vi "beginning_sound.vi"() -> ()   [LabVIEW 2019]
uses:
  <vilib>/sound2/lvsound2.llb/Sound Data Format.ctl
  <vilib>/sound2/lvsound2.llb/Sampling Mode.ctl
  <vilib>/sound2/lvsound2.llb/Sound Output Set Volume (Single).vi
  <vilib>/sound2/lvsound2.llb/Sound Output Write (DBL Single).vi
panel:
  out "sound":dbl
  in  "stop":bool
  in  "frequency":dbl
  in  "volume":dbl(slide) scale=0.0..100.0
  out "Waveform Chart":waveform(dbl)(graph)
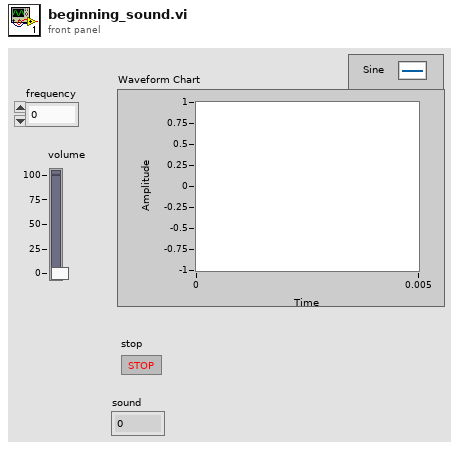
[diagram p1: front panel]
types:
  T1 = typedef "Sampling Mode.ctl" = i32
  T2 = typedef "Sound Data Format.ctl" = cluster{"sample rate (S/s)":dbl, "number of channels":i32, "bits per sample":i32}
  T3 = typedef "Sound Output Task ID.ctl" = u32
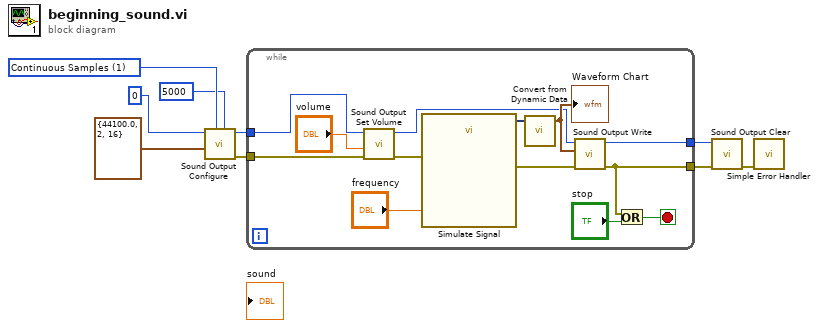
[diagram p0: block diagram]
diagram:
  w7 = T1 1 items=["Finite Samples", "Continuous Samples"] ("sample mode")
  n1 = call <vilib>:"Sound Output Configure.vi"("number of samples/ch"=5000, "sample mode"=w7, "sound format"=T2 {"sample rate (S/s)"=44100.0, "number of channels"=2, "bits per sample"=16}, "device ID"=u32 0) -> ("error out"=w5:errorcluster, "task ID"=w4:T3)  [unwired: 6 in]
  n2 = while {
    tunnel: w5 -> [w19]
    tunnel: w4 -> [w17]
    tunnel: [w11] -> w2
    tunnel: [w10] -> w3
    stop <- w21 stop-if-true
    n3 = call-poly <vilib>:"Sound Output Set Volume.vi"("error in (no error)"=w19, "volume"="volume", "task ID"=w17) -> ("error out"=w16:errorcluster, "task ID out"=w12:T3)  [unwired: 7 in]
    n4 = call "Simulate Signal"("Frequency"="frequency", "error in (no error)"=w16) -> ("Sine"=w15:dynamicdata, "error out"=w14:errorcluster)  [unwired: 12 in]
    n5 = call "Convert from Dynamic Data"("Dynamic Data Type"=w15) -> ("Waveform"=w13:waveform(dbl))  [unwired: 3 in]
    "Waveform Chart" <- w13
    n6 = call-poly <vilib>:"Sound Output Write.vi"("error in (no error)"=w14, "data"=w13, "task ID"=w12) -> ("error out"=w11:errorcluster, "task ID out"=w10:T3)  [unwired: 7 in]
    n7 = Or(x=w11, y="stop") -> (x .or. y?=w21:bool)
  }
  n8 = call <vilib>:"Sound Output Clear.vi"("error in (no error)"=w2, "task ID"=w3) -> ("error out"=w1:errorcluster)  [unwired: 9 in]
  n9 = call <vilib>:"Simple Error Handler.vi"("error in (no error)"=w1) -> ()  [unwired: 4 in, 5 out]
